vi "ms_to_s_U8.vi"(4 "time in":u8 caption="time in [ms]") -> (1 "time out":u8 caption="time out [s]")   [LabVIEW 2017, in "GPTiming.lvlib"]
doc: "Divides <B>time in</B> by 1,000 to convert it from milliseconds to seconds.\n\nEven though its functionality is really simple this function is valuable as it documents your code much better than a raw division by 1,000.\n\nThis VI is inlined.\n\nSteen Schmidt\nGPower\n9/12 2013"
uses:
  GPTiming.lvlib
panel:
  # "Copyright © 2013\nGPower\nSee enclosed license file for terms and conditions"
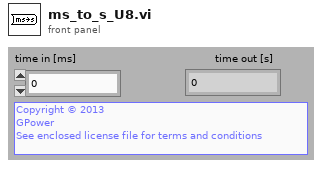
[diagram p1: front panel]
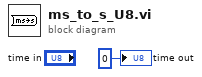
[diagram p0: block diagram]
diagram:
  "time out" <- u8 0 ("time out")
